vi "[HOST] UTILITIES Get Throughput.vi"(11 "Samples":u64[](array[numeric])) -> (3 "Throughput":dbl[](array[numeric]))   [LabVIEW 2016]
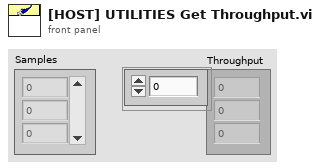
[diagram p1: front panel]
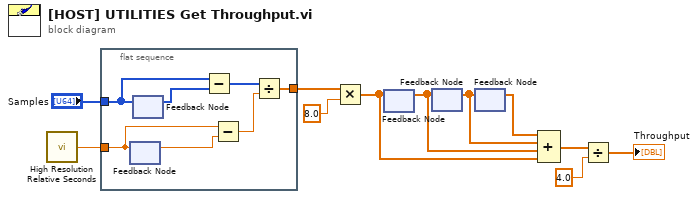
[diagram p0: block diagram]
diagram:
  n1 = call <vilib>:"High Resolution Relative Seconds.vi"() -> ("relative seconds"=w10:dbl)
  n2 = flat-sequence {
    tunnel: "Samples" -> [w17]
    tunnel: w10 -> [w15]
    tunnel: [w12] -> w9
    frame #0 {
      n3 = feedback #1() -> (w14:dbl)  [unwired: 1 in]
      n4 = feedback-in #1(w15) -> ()
      n5 = feedback #2() -> (w18:u64[])  [unwired: 1 in]
      n6 = feedback-in #2(w17) -> ()
      n7 = Subtract(x=w17, y=w18) -> (x-y=w16:u64[])
      n8 = Subtract(x=w15, y=w14) -> (x-y=w13:dbl)
      n9 = Divide(x=w16, y=w13) -> (x/y=w12:dbl[])
    }
  }
  n10 = Multiply(x=w9, y=8.0) -> (x*y=w4:dbl[])
  n11 = feedback-in #3(w4) -> ()
  n12 = feedback #3() -> (w5:dbl[])  [unwired: 1 in]
  n13 = feedback #4() -> (w6:dbl[])  [unwired: 1 in]
  n14 = feedback-in #4(w5) -> ()
  n15 = feedback #5() -> (w7:dbl[])  [unwired: 1 in]
  n16 = feedback-in #5(w6) -> ()
  n17 = Compound Arithmetic op=ADD(w7, w6, w5, w4) -> (w3:dbl[])
  n18 = Divide(x=w3, y=4.0) -> (x/y=→"Throughput":dbl[])
